vi "Init.vi"(8 "error in (no error)":errorcluster) -> (0 "error out":errorcluster, 3 "Distr uS Map ref out":refnum<data-value>)   [LabVIEW 2026, in "TALOS.lvlib" / "Classes.lvlib" / "Distributed uService Map.lvclass"]
uses:
  Distributed uService Map.lvclass
  Distributed uService Map.lvclass/Distributed uService Map.ctl
  Ancestor/Ancestor/Ancestor.lvclass/Ancestor.ctl
  Support VIs/Generate Error.vi
  FGV/Error Memory/Get Error Description.vi
  Support VIs/Get PC name.vi
  Ancestor/Ancestor/Read ID.vi
  Support VIs/Get Class Name.vi
  <vilib>/Utility/error.llb/Clear Errors.vi
  FGV/Error Memory/Error Memory Core.vi
  <vilib>/AdvancedString/Delimited String to 1D String Array (string).vi
  Support VIs/Circus Root Path.vi
  FGV/Error Memory/Error Crt Lvl checker.vi
  FGV/Error Memory/Error Memory Core.vi/40c8088d-b597-4017-91af-faa98e00292e.vi
  FGV/Error Memory/Error Memory Core.vi/d4a3ab98-063c-4e44-b43d-fbdcfe6c2be2.vi
  Support VIs/Global Memory.vi
  <vilib>/Utility/LVClass/Get LV Class Name.vi
  Support VIs/Is in Packed Library.vi
  Support VIs/TALOS Root path.vi
  Support VIs/Read CSV worksheet.vi
  Support VIs/Global Constants.vi
  <vilib>/Utility/error.llb/General Error Handler.vi
  Support VIs/Error Log.vi
  Ancestor/Ancestor/Ancestor.lvclass
  <vilib>/Comparison/Equal/Equal Functor/Equal Functor.lvclass
  TALOS.lvlib
  <vilib>/Utility/error.llb/Trim Whitespace (string).vi
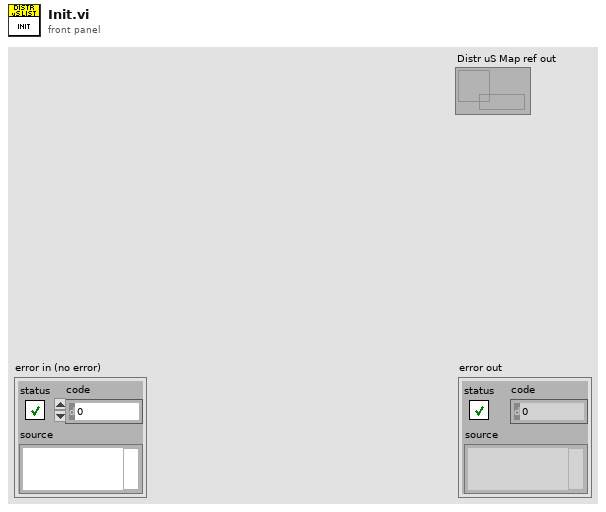
[diagram p1: front panel]
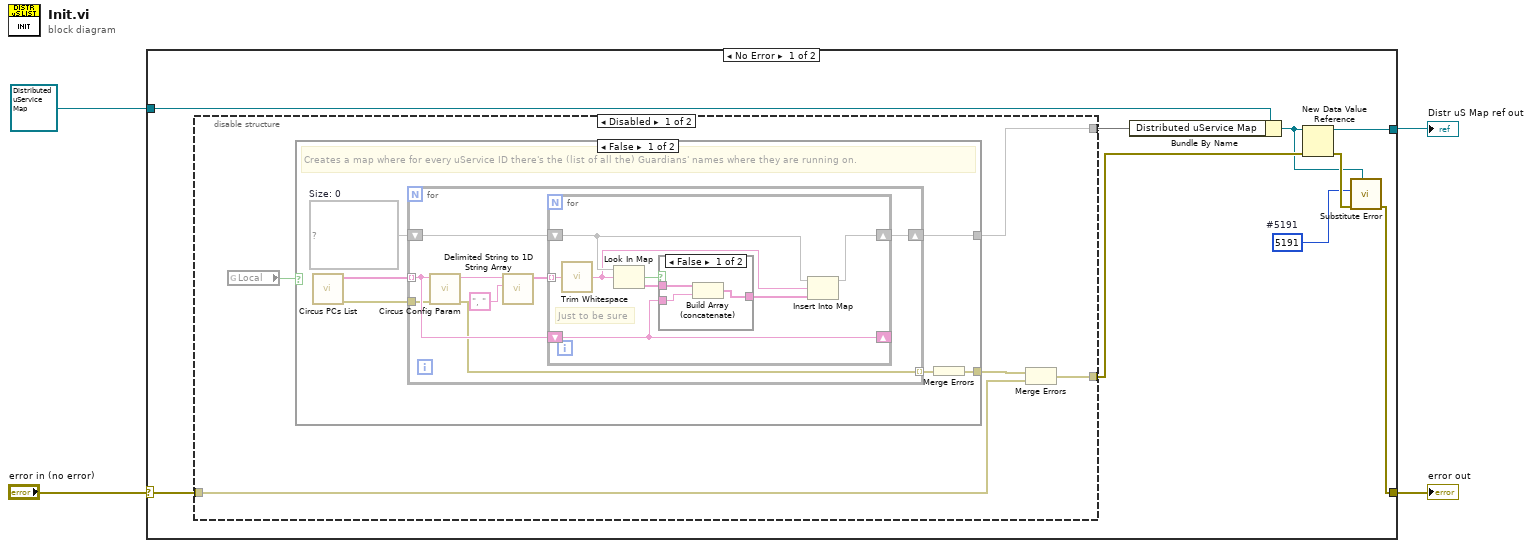
[diagram p0: block diagram]
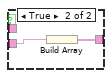
[diagram p2: hidden frame]
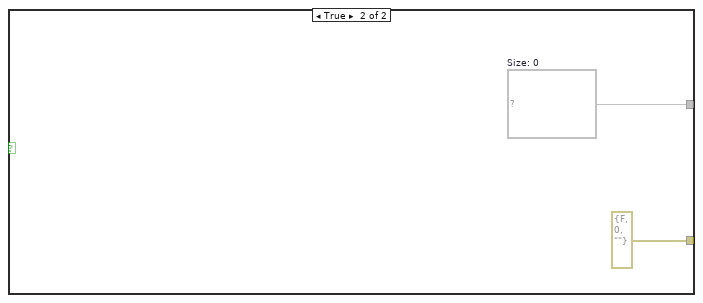
[diagram p3: hidden frame]
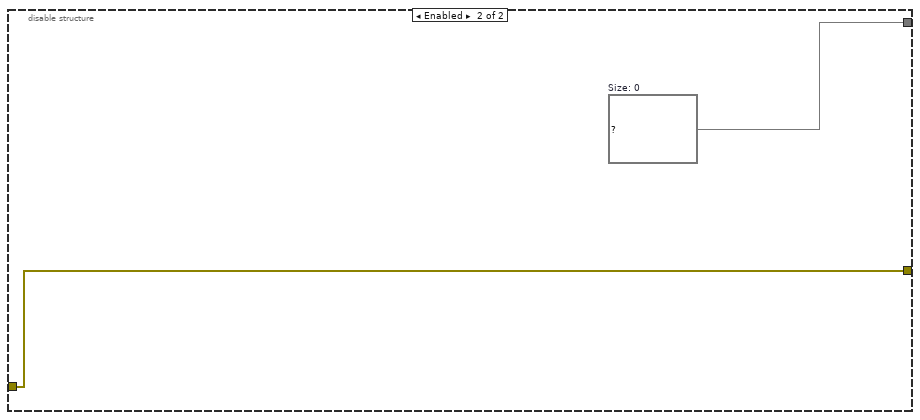
[diagram p4: hidden frame]
diagram:
  n1 = case shown="No Error" "error in (no error)" {
    selector: "error in (no error)" -> [w13 w50]
    tunnel: [w10 w50] -> w2
    tunnel: [w6 _] -> w1
    tunnel: refnum<class "Distributed uService Map.lvclass"> refnum ("Distributed uService Map in") -> [w12 _]
    frame No Error {
      w5 = 5191  # #5191
      n2 = disable-structure shown="Disabled" {
        disable-tunnel: w13 -> [w18 w49]
        disable-tunnel: [w17 w48] -> w11
        disable-tunnel: [w16 w49] -> w9
        frame Disabled {
          n3 = global read "Global Constants.vi" "Local"() -> (w14:bool)
          n4 = case shown="False" w14 {
            tunnel: [w23 w47] -> w17
            tunnel: [w20 errorcluster {"status"=FALSE, "code"=0, "source"=""} ("error IO")] -> w15
            frame False {
              w19 = map{string, string[]} {}  # Size: 0
              # "Creates a map where for every uService ID there's the (list of all the) Guardians' names where they are running on."
              n5 = call "Circus PCs List.vi"() -> ("error out"=w22:errorcluster, "PC List out"=w24:string[])  [unwired: 10 in]
              n6 = for {
                tunnel: w24 -> [w27] mode=indexing
                shift-right: [w28] -> w23
                shift-left: w19 -> [w29]
                tunnel: w22 -> [w26]
                tunnel: [w25] -> w21 mode=indexing
                n7 = call "Circus Config Param.vi"("error in (no error)"=w26, "Parameter Name"=w27) -> ("error out"=w25:errorcluster, "Value"=w30:string)  [unwired: 8 in]
                n8 = call-poly <vilib>:"Delimited String to 1D String Array.vi"("delimiter"=", ", "delimited string"=w30) -> ("string array"=w31:string[])  [unwired: 9 in]
                n9 = for {
                  tunnel: w31 -> [w40] mode=indexing
                  shift-right: [w36] -> w28
                  shift-left: w29 -> [w37]
                  shift-right: [w38] -> _
                  shift-left: w27 -> [w38]
                  # "Just to be sure"
                  n10 = call-poly <vilib>:"Trim Whitespace.vi"("string"=w40) -> ("trimmed string"=w35:string)  [unwired: 1 in]
                  n11 = Look In Map(map=w37, key=w35) -> (key not found?=w39:bool, value=w33:string[])  [unwired: 1 in]
                  n12 = case shown="False" w39 {
                    tunnel: w38 -> [w42 w45]
                    tunnel: [w41 w44] -> w34
                    tunnel: w33 -> [w43 _]
                    frame False {
                      n13 = Build Array (concatenate)(w43, w42) -> (w41:string[])
                    }
                    frame True {
                      n14 = Build Array(w45) -> (w44:string[])
                    }
                  }
                  n15 = Insert Into Map(map in=w37, key=w35, value=w34) -> (map out=w36:map{string, string[]})  [unwired: 2 out]
                }
              }
              n16 = Merge Errors(w21) -> (w20:errorcluster)
            }
            frame True {
              w47 = map{string, string[]} {}  # Size: 0
            }
          }
          n17 = Merge Errors(w15, w18) -> (w16:errorcluster)
        }
        frame Enabled {
          w48 = map{string, string[]} {}  # Size: 0
        }
      }
      n18 = Bundle By Name(cluster=w12, "Distributed uService Map"=w11) -> (w7:refnum<class "Distributed uService Map.lvclass">)
      n19 = New Data Value Reference(data value=w7, error in=w9) -> (data value reference=w6:refnum<data-value>, error out=w8:errorcluster)
      n20 = call "Substitute Error.vi"("LabVIEW Object"=w7, "error in (no error)"=w8, "Error Code"=w5) -> ("error out"=w10:errorcluster)  [unwired: 8 in]
    }
    frame Error {
    }
  }
  "error out" <- w2
  "Distr uS Map ref out" <- w1
